vi "Is Data Ready.vi"(8 "error in (no error)":errorcluster, 11 "Pulse Driver in":refnum<class "Pulse Driver.lvclass">) -> (0 "error out":errorcluster, 1 "Data ready":bool, 2 "Availiable Samples":u32, 3 "Pulse Driver out":refnum<class "Pulse Driver.lvclass">)   [LabVIEW 2015]
uses:
  Pulse Driver.lvclass
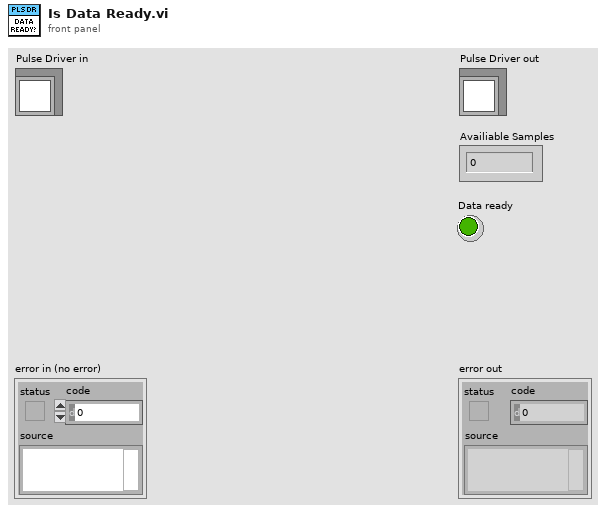
[diagram p1: front panel]
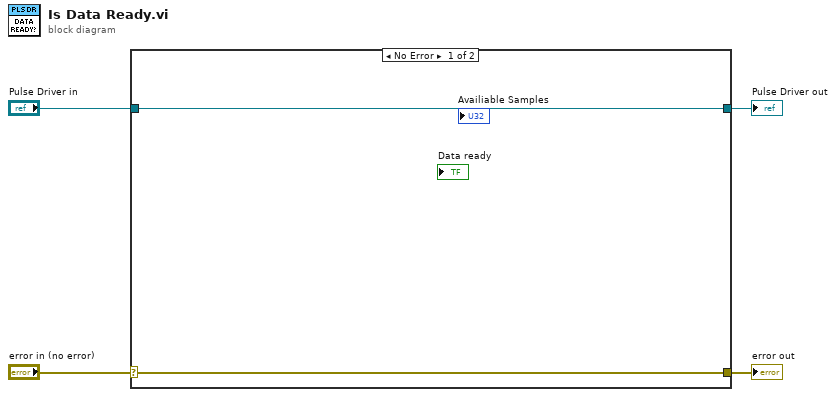
[diagram p0: block diagram]
diagram:
  n1 = case shown="No Error" "error in (no error)" {
    selector: "error in (no error)" -> [w5 w8]
    tunnel: [w5 w8] -> w3
    tunnel: [w6 w7] -> w1
    tunnel: "Pulse Driver in" -> [w6 w7]
    frame No Error {
    }
    frame Error {
    }
  }
  "error out" <- w3
  "Pulse Driver out" <- w1
